vi "RecordingParameterName.vi"(0 "StepMotor in":refnum<class "StepMotor.lvclass">, 11 "error in (no error)":errorcluster) -> (4 "StepMotor out":refnum<class "StepMotor.lvclass">, 15 "error out":errorcluster)   [LabVIEW 2010, in "StepMotor.lvclass"]
doc: "Запись праметра по имени в СПШ."
uses:
  StepMotor.lvclass
  StepMotor.lvclass/StepMotor.ctl
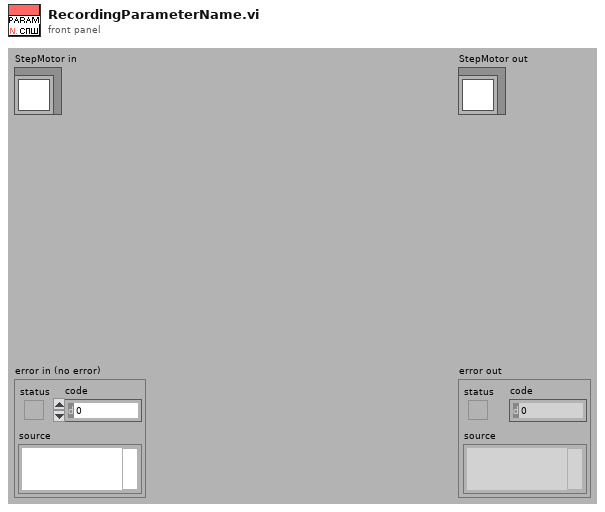
[diagram p1: front panel]
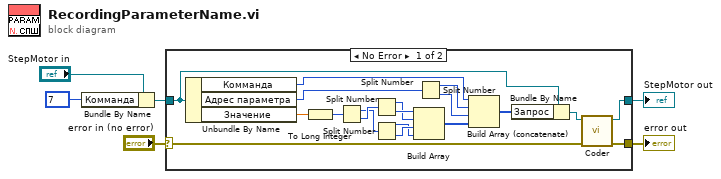
[diagram p0: block diagram]
diagram:
  n1 = Bundle By Name(cluster="StepMotor in", "Комманда"=u8 7 ("Numeric")) -> (w3:refnum<class "StepMotor.lvclass">)
  n2 = case shown="No Error" "error in (no error)" {
    selector: "error in (no error)" -> [w21 w27]
    tunnel: [w22 w26] -> w5
    tunnel: w3 -> [w16 w26]
    tunnel: [w20 w27] -> w1
    frame No Error {
      n3 = Unbundle By Name(w16) -> ("Комманда"=w17:u8, "Адрес параметра"=w25:u16, "Значение"=w15:dbl)
      n4 = To Long Integer(number=w15) -> (32bit integer=w11:i32)
      n5 = Split Number(x=w11) -> (hi(x)=w7:u16, lo(x)=w8:u16)
      n6 = Split Number(x=w8) -> (hi(x)=w9:u8, lo(x)=w10:u8)
      n7 = Split Number(x=w7) -> (hi(x)=w13:u8, lo(x)=w14:u8)
      n8 = Build Array(w10, w9, w14, w13) -> (w12:u8[])
      n9 = Split Number(x=w25) -> (hi(x)=w19:u8, lo(x)=w18:u8)
      n10 = Build Array (concatenate)(w17, w19, w18, w12) -> (w24:u8[])
      n11 = Bundle By Name(cluster=w16, "Запрос"=w24) -> (w23:refnum<class "StepMotor.lvclass">)
      n12 = call "Coder.vi"("error in (no error)"=w21, "StepMotor in"=w23) -> ("error out"=w20:errorcluster, "StepMotor out"=w22:refnum<class "StepMotor.lvclass">)  [unwired: 8 in]
    }
    frame Error {
    }
  }
  "error out" <- w1
  "StepMotor out" <- w5
